vi "notify_listeners.vi"(7 "force sending?":bool, 8 "error in (no error)":errorcluster, 9 "image finished?":bool, 10 "image (channels)":refnum<class "Image.lvclass">[](array[class]), 11 "GenericImageAssembler in":refnum<class "GenericImageAssembler.lvclass">) -> (0 "error out":errorcluster, 3 "GenericImageAssembler out":refnum<class "GenericImageAssembler.lvclass">)   [LabVIEW 2010]
uses:
  type_enum.ctl
  GenericImageAssembler.lvclass
  common/classes/GenericToplevelComponent/GenericToplevelComponent/GenericToplevelComponent.lvclass
  common/classes/Image/Image/Image.lvclass
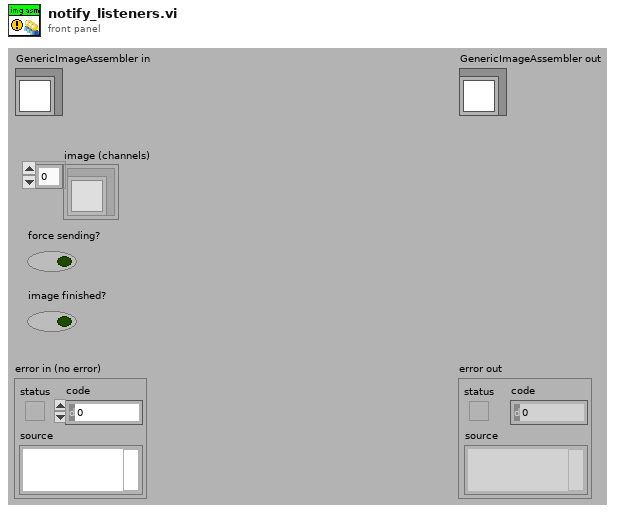
[diagram p1: front panel]
types:
  T1 = typedef "GenericImageAssembler.lvclass/type_enum.ctl" = enum16{"every step", "finalised images"}
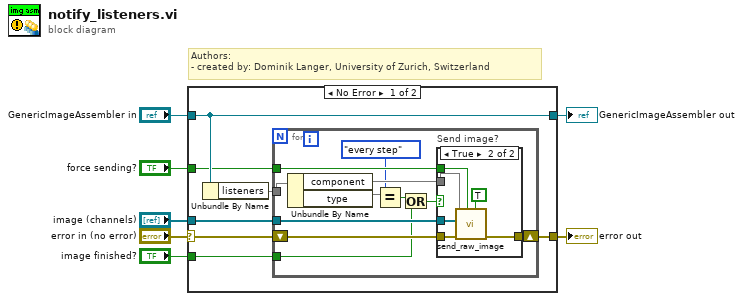
[diagram p0: block diagram]
diagram:
  # "Authors: \n- created by: Dominik Langer, University of Zurich, Switzerland"
  n1 = case shown="No Error" "error in (no error)" {
    selector: "error in (no error)" -> [w13 w34]
    tunnel: [w12 w34] -> w6
    tunnel: [w14 w33] -> w4
    tunnel: "GenericImageAssembler in" -> [w14 w33]
    tunnel: "image (channels)" -> [w10 _]
    tunnel: "force sending?" -> [w9 _]
    tunnel: "image finished?" -> [w8 _]
    frame No Error {
      n2 = Unbundle By Name(w14) -> ("listeners"=w11)
      n3 = for {
        shift-right: [w24] -> w12
        shift-left: w13 -> [w25]
        tunnel: w11 -> [w21]
        tunnel: w10 -> [w23]
        tunnel: w9 -> [w22]
        tunnel: w8 -> [w16]
        n4 = Unbundle By Name(w21) -> ("component"=w20, "type"=w19)
        n5 = Equal?(x=type_enum."every step" ("type"), y=w19) -> (x = y?=w17:bool)
        n6 = Or(x=w17, y=w16) -> (x .or. y?=w15:bool)
        n7 = case "Send image?" shown="True" w15 {
          tunnel: w25 -> [w26 w32]
          tunnel: [w26 w31] -> w24
          tunnel: w23 -> [_ w30]
          tunnel: w22 -> [_ w29]
          tunnel: w20 -> [_ w27]
          frame False {
          }
          frame True {
            n8 = call-dynamic "send_raw_image.vi"("send copy?"=TRUE, "enforce sending?"=w29, "error in (no error)"=w32, "image (channels)"=w30, "GenericToplevelComponent in"=w27) -> ("error out"=w31:errorcluster)  [unwired: 4 in, 2 out]
          }
        }
      }
    }
    frame Error {
    }
  }
  "error out" <- w6
  "GenericImageAssembler out" <- w4
